vi "Perform Action.vi"(7 "Target Ident":string, 8 "Error In":errorcluster, 10 "Input":variant, 11 "reference in":refnum<class "Measure and Stimulus Subsystems.lvclass">) -> (0 "Error Out":errorcluster, 2 "Output":variant, 3 "reference out":refnum<class "Measure and Stimulus Subsystems.lvclass">)   [LabVIEW 2023, in "HAL GOOP4.lvlib" / "Measure and Stimulus Subsystems.lvclass"]
uses:
  Measure and Stimulus Subsystems.lvclass
  <vilib>/Utility/error.llb/Error Cluster From Error Code.vi
  <vilib>/ErrorRing/Error Ring.xnode
  Virtual Instrument Base/Virt Instr Base.lvclass
  Measure and Stimulus Subsystems.lvclass/Measure and Stimulus Subsystems.ctl
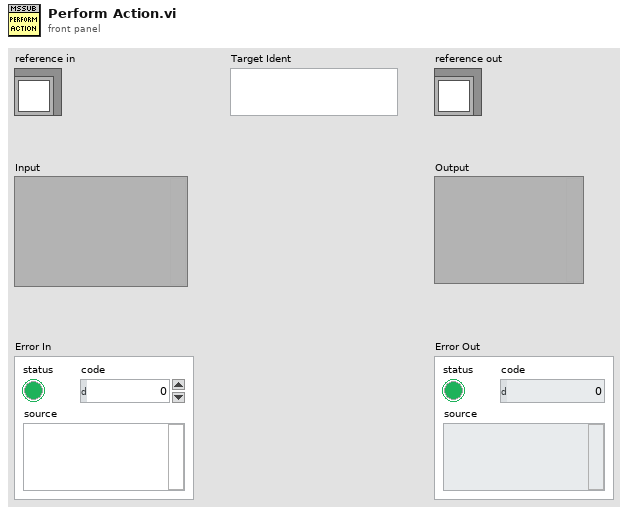
[diagram p1: front panel]
types:
  T1 = typedef "HAL GOOP4.lvlib/Measure and Stimulus Subsystems.lvclass/ObjectAttributes.ctl" = cluster{"Virt Instr":map{string, refnum<class "Virt Instr Base.lvclass">}, "Phys Instr":map{string, cluster{"Instrument":refnum<class "Instrument.lvclass">, "Ref Count":u8}}}
  T2 = map{string, refnum<class "Virt Instr Base.lvclass">}
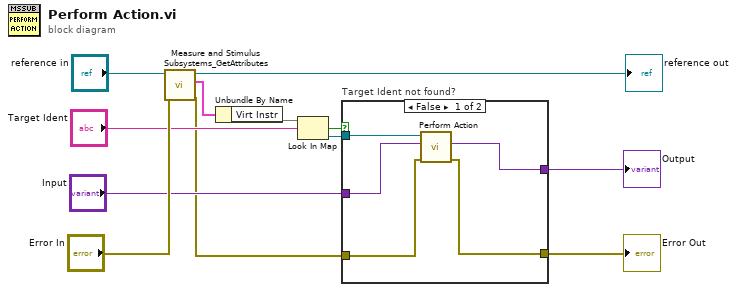
[diagram p0: block diagram]
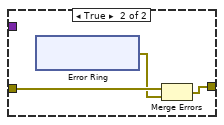
[diagram p2: hidden frame]
diagram:
  n1 = call "Measure and Stimulus Subsystems_GetAttributes.vi"("Error In"="Error In", "reference in"="reference in") -> ("Error Out"=w1:errorcluster, "Data"=w7:T1, "reference out"=→"reference out":refnum<class "Measure and Stimulus Subsystems.lvclass">)  [unwired: 6 in, 1 out]
  n2 = Unbundle By Name(w7) -> ("Virt Instr"=w6:T2)
  n3 = Look In Map(map=w6, key="Target Ident") -> (key not found?=w4:bool, value=w3:refnum<class "Virt Instr Base.lvclass">)  [unwired: 1 in]
  n4 = case "Target Ident not found?" shown="False" w4 {
    tunnel: w1 -> [w14 w20]
    tunnel: w3 -> [w17 _]
    tunnel: [w13 w18] -> w8
    tunnel: [w16 _] -> w9
    tunnel: "Input" -> [w15 _]
    frame False {
      n5 = call-dynamic "Perform Action.vi"("error in (no error)"=w14, "Input"=w15, "Virt Instrument Base in"=w17) -> ("error out"=w13:errorcluster, "Output"=w16:variant)  [unwired: 6 in, 1 out]
    }
    frame True {
      n6 = xnode "Error Ring"() -> ("error out"=w19:errorcluster)
      n7 = Merge Errors(w20, w19) -> (w18:errorcluster)
    }
  }
  "Error Out" <- w8
  "Output" <- w9
